vi "different shapes.vi"() -> ()   [LabVIEW 2019]
uses:
  <vilib>/eio/EIONode/EIONode.xnode
  <vilib>/rvi/eio/common/nirviEmuTemplateMethod_errors.vi
  <vilib>/rvi/DataTransferAndStorage/Container/XNode/niFpgaContainer.xnode
  <vilib>/rvi/FIFO/Fifo_Resource/nirvififoEmulationRead.vi
  <vilib>/eio/EIOPropertyNode/EIOPropertyNode.xnode
  <vilib>/rvi/eio/common/nirviEmuTemplatePropertyGet_errors.vi
  <vilib>/rvi/eio/common/nirviEmuTemplatePropertyGet_noerrors.vi
  <vilib>/rvi/eio/common/nirviEmuTemplatePropertySet_errors.vi
  <vilib>/rvi/eio/common/nirviEmuTemplatePropertySet_noerrors.vi
  <vilib>/rvi/FIFO/Fifo_Resource/nirvififoEmulationWrite.vi
  <vilib>/rvi/interface/RandomDataEmulation/nirviRandomDataFpgaReadWriteTemplate.vi
panel:
  in  "Force_ST":sgl
  in  "shape":i16(ring) items=["Harmonic", "Sawtooth", "Quartic"]
  in  "1/Ycali":sgl
  out "Fy out/Ycorr":sgl
  in  "Enum":enum8{"No FB", "FB"}(ring)
  in  "MobX(px/V)":sgl
  in  "1/Xcali":sgl
  in  "Feedback parameters":T1
  in  "DX":sgl
  in  "Xmean":sgl
  in  "Frequency":u32=100000
  in  "Triangle wave":T2={"signal offset_X"=5.0, "Scale X"=0.0, "signal offset_Y"=5.0, "Scale Y"=0.0, "Phase Shift"=30}
  out "Fx out/Xcorr":sgl
  in  "Xoffset":sgl
  in  "Yoffset":sgl
  in  "sum_offset":sgl
  in  "Normalize signal":bool=TRUE
  in  "FB Time":u8=5 caption="Feedback loop time"
  out "Saveloop":u32
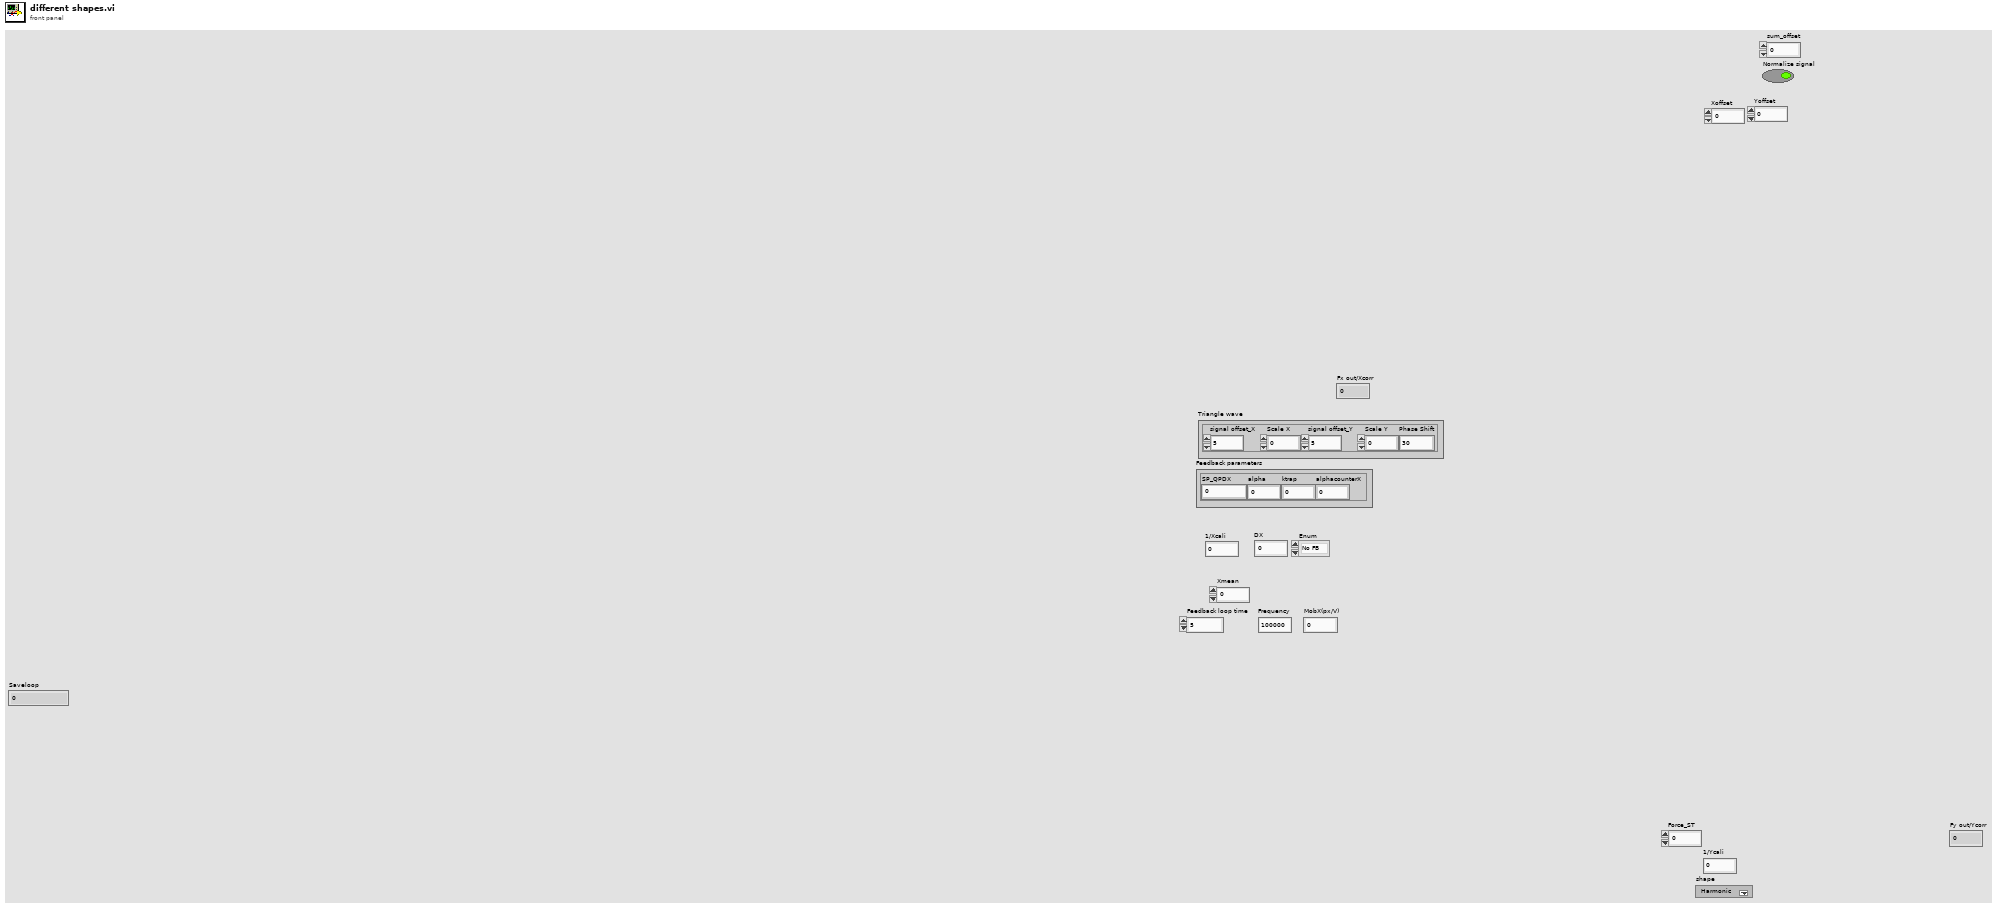
[diagram p1: front panel]
types:
  T1 = cluster{"SP_QPDX":sgl, "alpha":sgl, "ktrap":sgl, "alphacounterX":sgl}
  T2 = cluster{"signal offset_X":sgl, "Scale X":sgl, "signal offset_Y":sgl, "Scale Y":sgl, "Phase Shift":u32}
  T3 = enum8{"+/- 10 V", "+/- 5 V", "+/- 2 V", "+/- 1 V"}
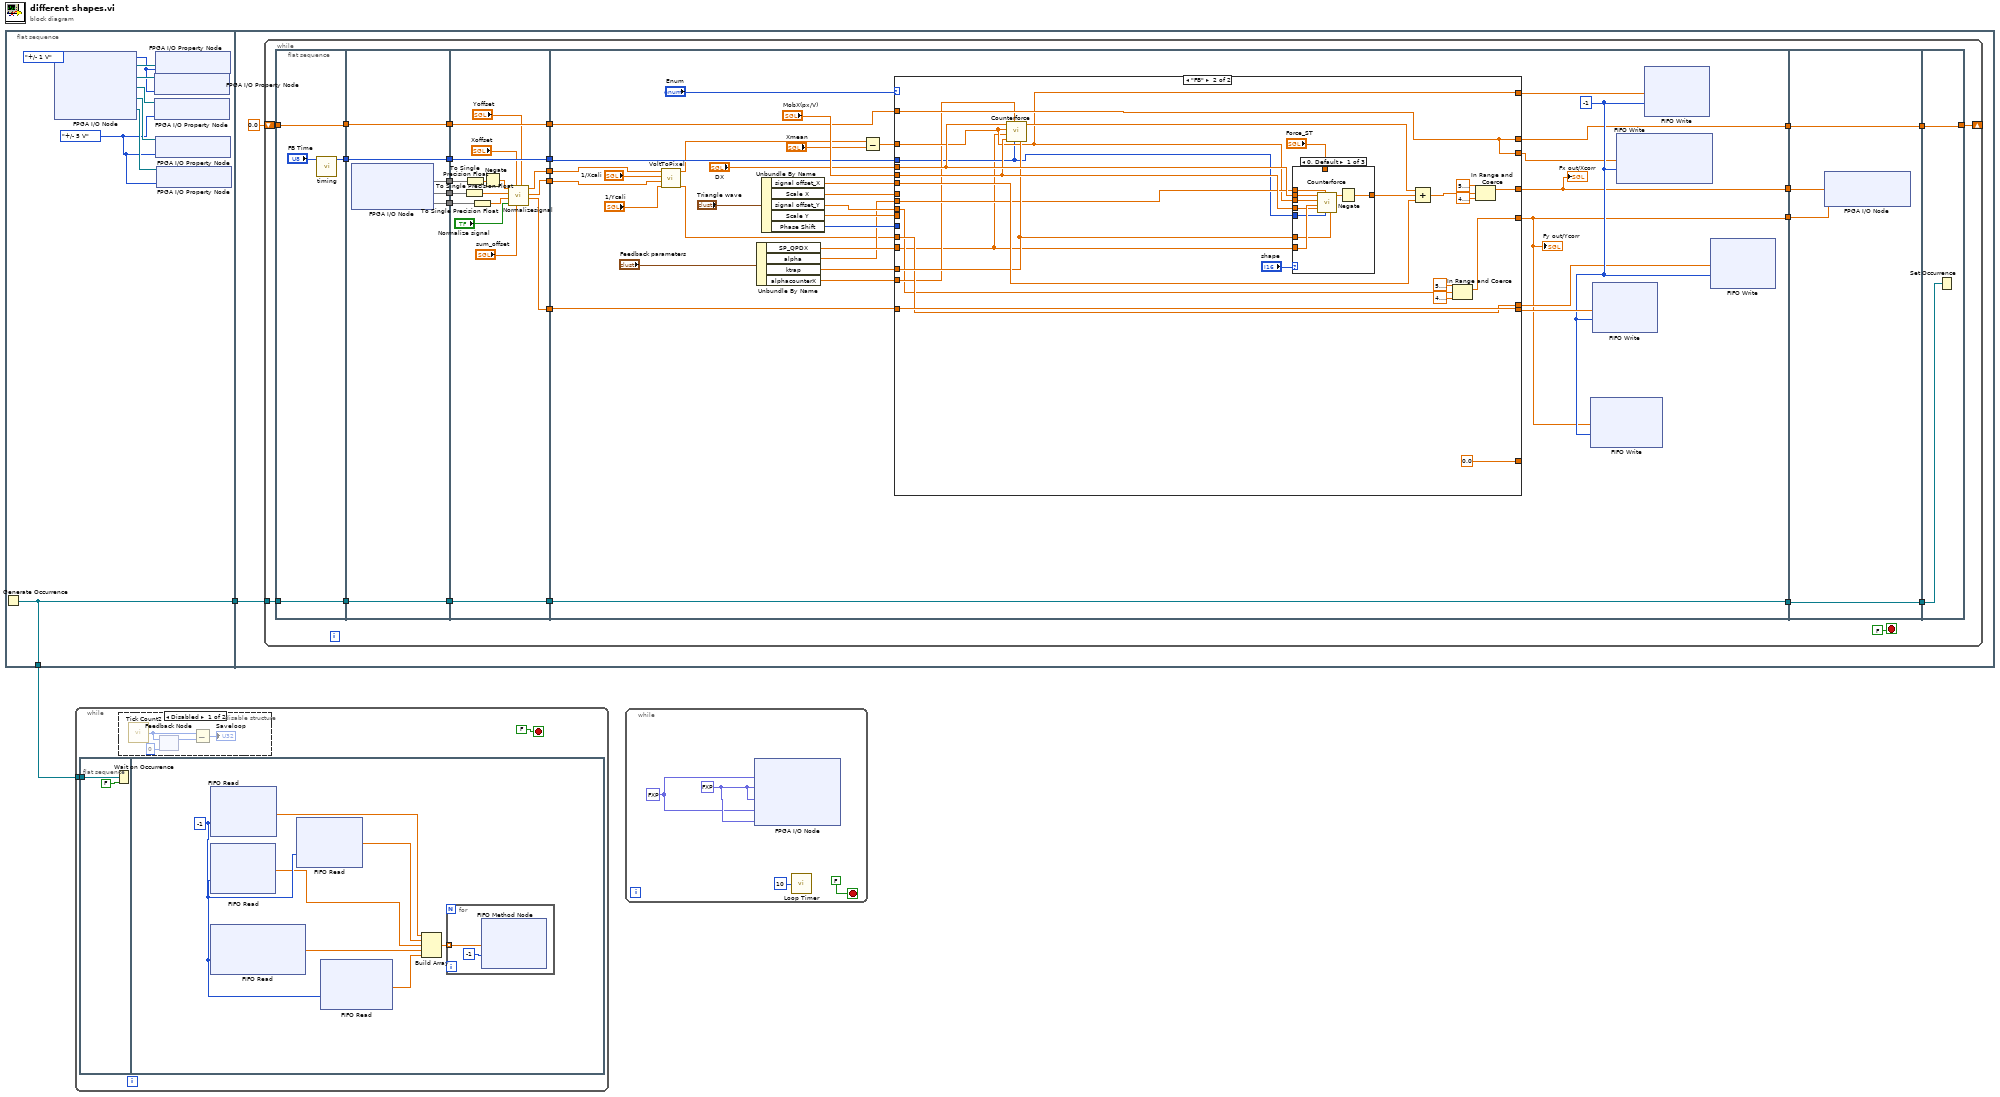
[diagram p0: block diagram]
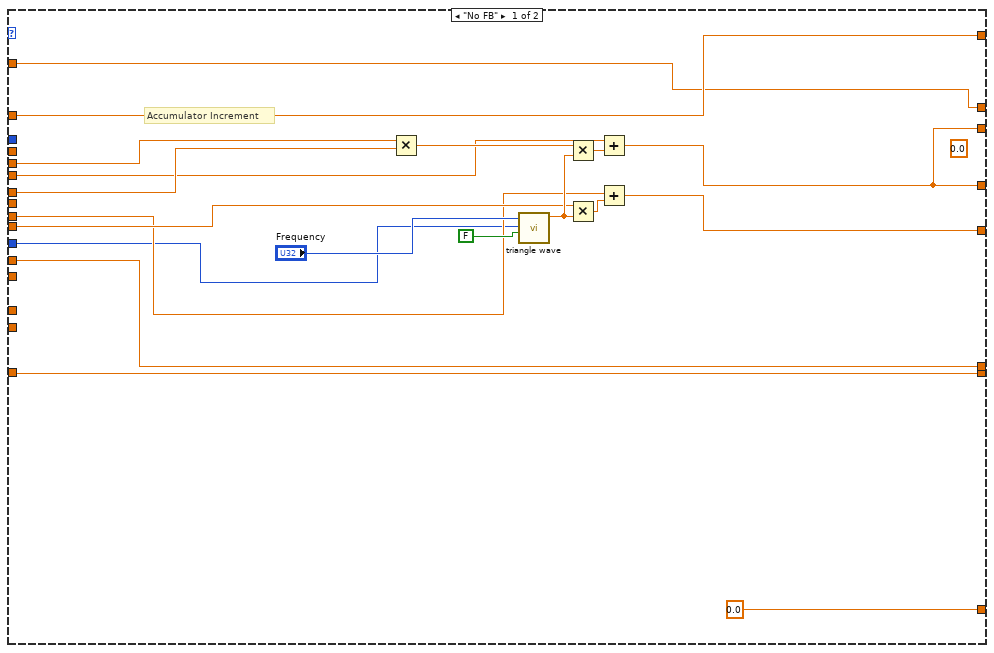
[diagram p2: hidden frame]
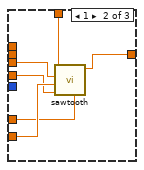
[diagram p3: hidden frame]
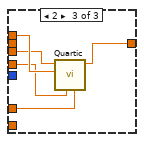
[diagram p4: hidden frame]
diagram:
  n1 = flat-sequence {
    tunnel: [w3] -> w2
    tunnel: [w3] -> w1
    tunnel: w2 -> [w12]
    frame #0 {
      w4 = T3."+/- 5 V" ("Voltage Range")
      w7 = T3."+/- 1 V" ("Voltage Range")
      n2 = Generate Occurrence() -> (w3:refnum<k4>)
      n3 = xnode "FPGA I/O Node"() -> ("FPGA I/O Out"=w10:refnum<k21>, "FPGA I/O Out"=w8:refnum<k21>, "FPGA I/O Out"=w9:refnum<k21>, "FPGA I/O Out"=w5:refnum<k21>, "FPGA I/O Out"=w6:refnum<k21>)  [unwired: 5 in, 5 out]
      n4 = xnode "FPGA I/O Property Node"("FPGA I/O In"=w8, "Voltage Range"=w7) -> ()  [unwired: 1 out]
      n5 = xnode "FPGA I/O Property Node"("FPGA I/O In"=w9, "Voltage Range"=w4) -> ()  [unwired: 1 out]
      n6 = xnode "FPGA I/O Property Node"("FPGA I/O In"=w10, "Voltage Range"=w7) -> ()  [unwired: 1 out]
      n7 = xnode "FPGA I/O Property Node"("FPGA I/O In"=w5, "Voltage Range"=w4) -> ()  [unwired: 1 out]
      n8 = xnode "FPGA I/O Property Node"("FPGA I/O In"=w6, "Voltage Range"=w4) -> ()  [unwired: 1 out]
    }
    frame #1 {
      n9 = while {
        tunnel: w12 -> [w25]
        shift-right: [w17] -> _
        shift-left: sgl 0.0 -> [w15]
        stop <- FALSE ("stop") stop-if-true
        n10 = flat-sequence {
          tunnel: [w40] -> w26
          tunnel: w25 -> [w39]
          tunnel: [w39] -> w24
          tunnel: [w38] -> w16
          tunnel: w15 -> [w38]
          tunnel: [w47] -> w36
          tunnel: [w46] -> w34
          tunnel: [w45] -> w32
          tunnel: [w44] -> w27
          tunnel: w26 -> [w44]
          tunnel: w24 -> [w43]
          tunnel: [w43] -> w23
          tunnel: w16 -> [w42]
          tunnel: [w42] -> w13
          tunnel: w36 -> [w54]
          tunnel: [w63] -> w35
          tunnel: w34 -> [w53]
          tunnel: [w62] -> w33
          tunnel: w32 -> [w51]
          tunnel: [w61] -> w31
          tunnel: [w64] -> w28
          tunnel: w27 -> [w64]
          tunnel: w23 -> [w60]
          tunnel: [w60] -> w22
          tunnel: [w58] -> w14
          tunnel: w13 -> [w58]
          tunnel: w35 -> [w95]
          tunnel: w33 -> [w68]
          tunnel: w31 -> [w94]
          tunnel: [w70] -> w30
          tunnel: [w66] -> w29
          tunnel: w28 -> [w96]
          tunnel: w22 -> [w89]
          tunnel: [w89] -> w20
          tunnel: [w84] -> w19
          tunnel: w14 -> [w83]
          tunnel: w29 -> [w165]
          tunnel: w30 -> [w166]
          tunnel: [w164] -> w21
          tunnel: w20 -> [w164]
          tunnel: w19 -> [w163]
          tunnel: [w163] -> w18
          tunnel: w21 -> [w168]
          tunnel: [w167] -> w17
          tunnel: w18 -> [w167]
          frame #0 {
            n11 = call "timing.vi"("Feedback loop time"="FB Time") -> ("Feedback Loop time"=w40:u32)  [unwired: 10 in]
          }
          frame #1 {
            n12 = xnode "FPGA I/O Node"() -> ("Connector1/AI2"=w47, "Connector1/AI4"=w46, "Connector1/AI5"=w45)  [unwired: 3 in, 3 out]
          }
          frame #2 {
            n13 = To Single Precision Float(number=w53) -> (single precision float=w52:sgl)
            n14 = To Single Precision Float(number=w54) -> (single precision float=w49:sgl)
            n15 = To Single Precision Float(number=w51) -> (single precision float=w50:sgl)
            n16 = Negate(x=w49) -> (-x=w48:sgl)
            n17 = call "Normalizesignal.vi"("Yoffset"="Yoffset", "sum_offset"="sum_offset", "Xoffset"="Xoffset", "Normalize signal"="Normalize signal", "Sum"=w50, "Y"=w52, "X"=w48) -> ("Sum"=w61:sgl, "Y"=w62:sgl, "X"=w63:sgl)  [unwired: 2 in]
          }
          frame #3 {
            w85 = -1 ("Timeout")
            n18 = call "VoltToPixel.vi"("1/(QPDY/px)"="1/Ycali", "Normalized Y"=w68, "1/(QPDX/px)"="1/Xcali", "Normalized X"=w95) -> ("Ypx"=w65:sgl, "Xpx"=w88:sgl)  [unwired: 6 in]
            n19 = Unbundle By Name("Feedback parameters") -> ("SP_QPDX"=w75:sgl, "alpha"=w72:sgl, "ktrap"=w73:sgl, "alphacounterX"=w74:sgl)
            n20 = Unbundle By Name("Triangle wave") -> ("signal offset_X"=w79:sgl, "Scale X"=w81:sgl, "signal offset_Y"=w78:sgl, "Scale Y"=w80:sgl, "Phase Shift"=w77:u32)
            n21 = Subtract(x=w88, y="Xmean") -> (x-y=w92:sgl)
            n22 = case shown="\"FB\"" "Enum" {
              tunnel: w92 -> [w115 w127]
              tunnel: [w99 w139] -> w70
              tunnel: [w109 w124] -> w66
              tunnel: [w115 w127] -> w91
              tunnel: [w117 w131] -> w90
              tunnel: w94 -> [w117 w131]
              tunnel: w65 -> [w116 w130]
              tunnel: [w116 w130] -> w71
              tunnel: "MobX(px/V)" -> [w108 w141]
              tunnel: w96 -> [_ w121]
              tunnel: "DX" -> [_ w142]
              tunnel: [sgl 0.0 ("f") sgl 0.0 ("f")] -> _
              tunnel: [w107 w132] -> w84
              tunnel: w83 -> [w107 w132]
              tunnel: w81 -> [w105 _]
              tunnel: w80 -> [w104 _]
              tunnel: w79 -> [w103 w138]
              tunnel: w78 -> [w102 w120]
              tunnel: w77 -> [w101 _]
              tunnel: w75 -> [_ w119]
              tunnel: w74 -> [_ w122]
              tunnel: w73 -> [_ w137]
              tunnel: w72 -> [_ w136]
              tunnel: [w99 w132] -> w69
              frame "No FB" {
                (unwired) sgl 0.0 ("f")
                # "Accumulator Increment"
                n23 = Multiply(x=w108, y=w105) -> (x*y=w113:sgl)
                n24 = call "triangle wave.vi"("Reset Accumulator_TW"=FALSE, "phase shift"=w101, "Frequency"="Frequency") -> ("Tri wave out"=w110:sgl)  [unwired: 8 in]
                n25 = Multiply(x=w113, y=w110) -> (x*y=w112:sgl)
                n26 = Multiply(x=w104, y=w110) -> (x*y=w114:sgl)
                n27 = Add(x=w103, y=w112) -> (x+y=w99:sgl)
                n28 = Add(x=w102, y=w114) -> (x+y=w109:sgl)
              }
              frame "FB" {
                n29 = call "Counterforce.vi"("ktrap"=w137, "Ts"=w121, "alphacounterX"=w122, "mobX(px/V)"=w141, "SP_X"=w119, "Xpx"=w127, "Dx"=w142) -> ("counter Force"=w140:sgl)  [unwired: 2 in, 2 out]
                n30 = case shown="0, Default" "shape" {
                  tunnel: w142 -> [w148 _ _]
                  tunnel: w141 -> [w145 w155 w159]
                  tunnel: w137 -> [w143 w154 w160]
                  tunnel: w136 -> [w149 _ w162]
                  tunnel: [w150 w153 w158] -> w129
                  tunnel: w127 -> [w147 w157 w161]
                  tunnel: w121 -> [w144 _ _]
                  tunnel: w119 -> [w146 w156 _]
                  tunnel: "Force_ST" -> [_ w152 _]
                  frame 0, Default {
                    n31 = call "Counterforce.vi"("ktrap"=w143, "Ts"=w144, "alphacounterX"=w149, "mobX(px/V)"=w145, "SP_X"=w146, "Xpx"=w147, "Dx"=w148) -> ("counter Force"=w151:sgl)  [unwired: 2 in, 2 out]
                    n32 = Negate(x=w151) -> (-x=w150:sgl)
                  }
                  frame 1 {
                    n33 = call "sawtooth.vi"("ktrap"=w154, "mobX(px/V)"=w155, "SP_X"=w156, "Xpx"=w157, "Force_ST"=w152) -> ("counter Force"=w153:sgl)  [unwired: 6 in]
                  }
                  frame 2 {
                    n34 = call "Quartic.vi"("ktrap"=w160, "mobX(px/V)"=w159, "alpha quartic"=w162, "Xpx"=w161) -> ("counter Force"=w158:sgl)  [unwired: 7 in]
                  }
                }
                n35 = Compound Arithmetic op=ADD(w140, w129, w138) -> (w135:sgl)
                n36 = In Range and Coerce(upper limit=sgl 5.1, x=w120, lower limit=sgl 4.9) -> (coerced(x)=w124:sgl)  [unwired: 1 out]
                n37 = In Range and Coerce(upper limit=sgl 5.1, x=w135, lower limit=sgl 4.9) -> (coerced(x)=w139:sgl)  [unwired: 1 out]
              }
            }
            "Fx out/Xcorr" <- w70
            "Fy out/Ycorr" <- w66
            n38 = xnode ("FIFO Write")("Element"=w66, "Timeout"=w85) -> ()  [unwired: 1 in, 2 out]
            n39 = xnode ("FIFO Write")("Element"=w90, "Timeout"=w85) -> ()  [unwired: 1 in, 2 out]
            n40 = xnode ("FIFO Write")("Element"=w69, "Timeout"=w85) -> ()  [unwired: 1 in, 2 out]
            n41 = xnode ("FIFO Write")("Element"=w91, "Timeout"=w85) -> ()  [unwired: 1 in, 2 out]
            n42 = xnode ("FIFO Write")("Element"=w71, "Timeout"=w85) -> ()  [unwired: 1 in, 2 out]
          }
          frame #4 {
            n43 = xnode "FPGA I/O Node"("Connector1/AO7"=w166, "Connector1/AO6"=w165) -> ()  [unwired: 2 in, 2 out]
          }
          frame #5 {
            n44 = Set Occurrence(w168) -> ()
          }
        }
      }
    }
  }
  n45 = while {
    tunnel: w1 -> [w169]
    stop <- FALSE stop-if-true
    n46 = flat-sequence {
      tunnel: w169 -> [w176]
      frame #0 {
        n47 = Wait on Occurrence(1:FALSE ("ignore previous (T)"), 2:w176) -> ()  [unwired: 1 in, 1 out]
      }
      frame #1 {
        w179 = -1 ("Timeout")
        n48 = xnode ("FIFO Read")("Timeout"=w179) -> ("Element"=w177:sgl)  [unwired: 1 in, 2 out]
        n49 = xnode ("FIFO Read")("Timeout"=w179) -> ("Element"=w180:sgl)  [unwired: 1 in, 2 out]
        n50 = xnode ("FIFO Read")("Timeout"=w179) -> ("Element"=w181:sgl)  [unwired: 1 in, 2 out]
        n51 = xnode ("FIFO Read")("Timeout"=w179) -> ("Element"=w178:sgl)  [unwired: 1 in, 2 out]
        n52 = xnode ("FIFO Read")("Timeout"=w179) -> ("Element"=w182:sgl)  [unwired: 1 in, 2 out]
        n53 = Build Array(w181, w178, w177, w180, w182) -> (w183:sgl[])
        n54 = for {
          tunnel: w183 -> [w185] mode=indexing
          n55 = xnode ("FIFO Method Node")("Element"=w185, "Timeout"=-1) -> ()  [unwired: 1 in, 2 out]
        }
      }
    }
    n56 = disable-structure shown="Disabled" {
      frame Disabled {
        n57 = call "Tick Count2"() -> ("Tick Count(uSec)"=w174:u32)
        n58 = feedback #1(u32 0 ("Tick Count(uSec)")) -> (w173:u32)
        n59 = feedback-in #1(w174) -> ()
        n60 = Subtract(x=w174, y=w173) -> (x-y=→"Saveloop":u32)
      }
      frame Enabled {
      }
    }
  }
  n61 = while {
    stop <- FALSE stop-if-true
    w186 = fxp<+,8,3> 2.5 ("Connector1/AO2")
    w187 = fxp<+,8,3> 5.0 ("Connector1/AO2")
    n62 = xnode "FPGA I/O Node"("Connector1/AO0"=w186, "Connector1/AO2"=w187, "Connector1/AO3"=w187, "Connector1/AO4"=w186, "Connector1/AO5"=w187) -> ()  [unwired: 5 in, 5 out]
    n63 = call "Loop Timer"("Count(uSec)"=u8 10) -> ()  [unwired: 1 out]
  }
